vi "Sensifier.vi"(11 "Array":string[](array[string])) -> (1 "Removed Strings":string[](array[string]), 2 "Has Errors?":bool, 3 "Sensed":string[](array[string]))   [LabVIEW 2014]
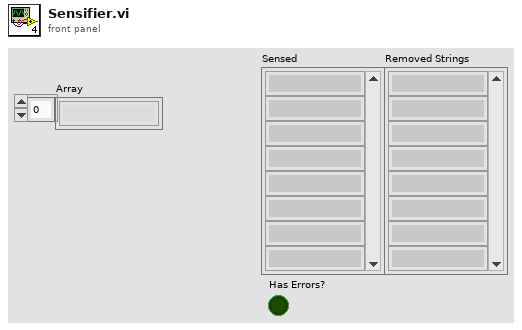
[diagram p1: front panel]
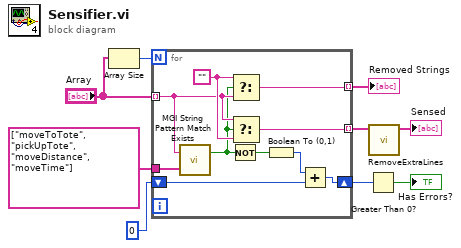
[diagram p0: block diagram]
diagram:
  n1 = Array Size(array="Array") -> (size(s)=w7:i32)
  n2 = for {
    N: w7 -> [_]
    tunnel: "Array" -> [w13] mode=indexing
    tunnel: string[] ["moveToTote", "pickUpTote", "moveDistance", "moveTime"] ("string array") -> [w19]
    tunnel: [w18] -> w5 mode=indexing
    shift-right: [w17] -> w4
    shift-left: i16 0 -> [w16]
    tunnel: [w12] -> w2 mode=indexing
    w14 = ""
    n3 = call <userlib>:"MGI String Pattern Match Exists.vi"("Patterns to Try"=w19, "String"=w13) -> ("Match Found"=w10:bool)  [unwired: 1 out]
    n4 = Not(x=w10) -> (.not. x?=w11:bool)
    n5 = Select(t=w14, s=w10, f=w13) -> (s? t:f=w12:string)
    n6 = Select(t=w13, s=w10, f=w14) -> (s? t:f=w18:string)
    n7 = Boolean To (0,1)(Boolean=w11) -> (0, 1=w15:i16)
    n8 = Add(x=w15, y=w16) -> (x+y=w17:i16)
  }
  "Removed Strings" <- w2
  n9 = Greater Than 0?(x=w4) -> (x > 0?=→"Has Errors?":bool)
  n10 = call "RemoveExtraLines.vi"("Sensed"=w5) -> ("Output"=→"Sensed":string[])  [unwired: 10 in]
